vi "Transform.vi"(8 "error in (no error)":errorcluster caption="entrée d'erreur (pas d'erreur)", 9 "y":string[][](array[string]), 10 "X":string[][](array[string]), 11 "KernelCenterer.lvclass":refnum<class "KernelCenterer.lvclass">) -> (0 "error out":errorcluster caption="sortie d'erreur", 2 "Data":T1, 3 "KernelCenterer.lvclass":refnum<class "KernelCenterer.lvclass">)   [LabVIEW 2020, in "KernelCenterer.lvclass"]
doc: "Center kernel matrix.\n\nReturns : \n\n- K_new : numpy array of shape [n_samples1, n_samples2]"
uses:
  KernelCenterer.lvclass
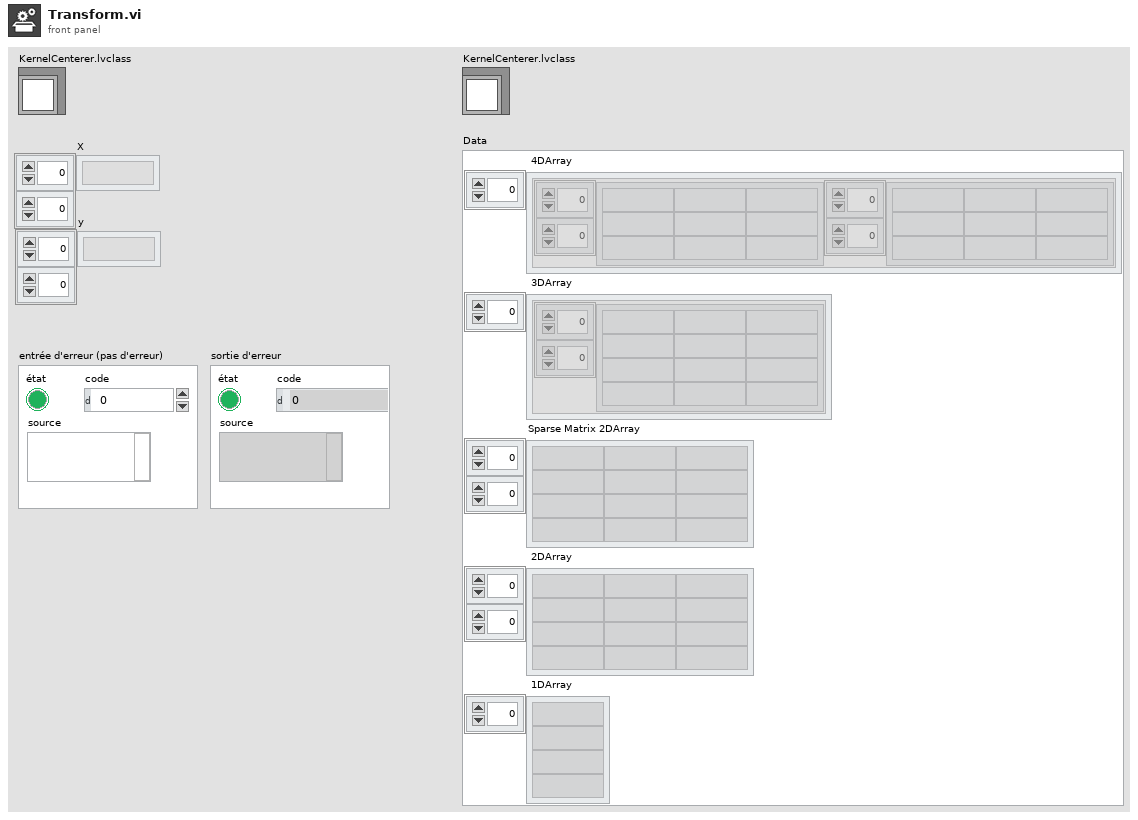
[diagram p1: front panel]
types:
  T1 = cluster{" 4DArray":cluster{"1":string[][], "2":string[][]}[], " 3DArray":cluster{"Tableau":string[][]}[], "Sparse Matrix 2DArray":string[][], " 2DArray":string[][], " 1DArray":string[]}
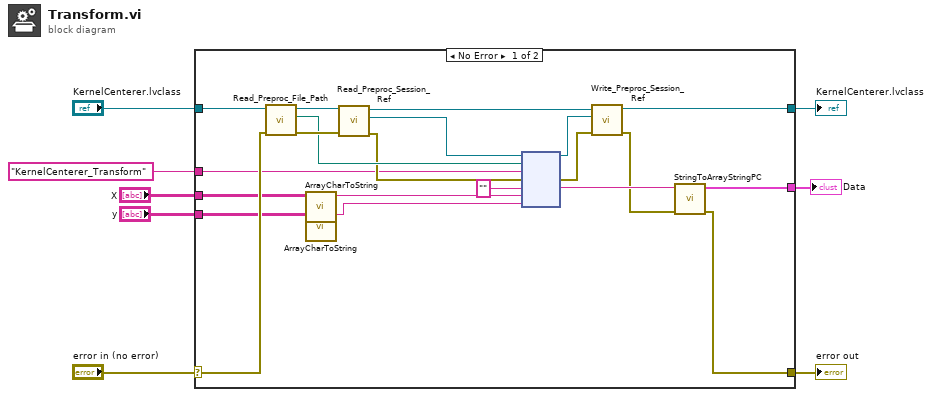
[diagram p0: block diagram]
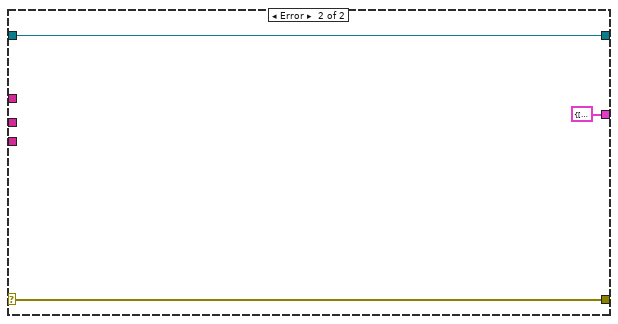
[diagram p2: hidden frame]
diagram:
  n1 = case shown="No Error" "error in (no error)" {
    selector: "error in (no error)" -> [w19 w32]
    tunnel: [w9 w32] -> w7
    tunnel: [w12 w31] -> w5
    tunnel: "KernelCenterer.lvclass" -> [w20 w31]
    tunnel: "KernelCenterer_Transform" ("Fonction") -> [w18 _]
    tunnel: [w10 T1 {" 4DArray"=[], " 3DArray"=[], "Sparse Matrix 2DArray"=[], " 2DArray"=[], " 1DArray"=[]} ("Data")] -> w1
    tunnel: "X" -> [w17 _]
    tunnel: "y" -> [w16 _]
    frame No Error {
      n2 = call-dynamic "Read_Preproc_File_Path.vi"("error in (no error)"=w19, "Python in"=w20) -> ("error out"=w28:errorcluster, "File_Path"=w25:path, "Python out"=w29:refnum<class "KernelCenterer.lvclass">)  [unwired: 7 in]
      n3 = call "ArrayCharToString.vi"("TAB"=w17) -> ("Instruction"=w15:string)  [unwired: 10 in]
      n4 = call "ArrayCharToString.vi"("TAB"=w16) -> ("Instruction"=w14:string)  [unwired: 10 in]
      n5 = call-dynamic "Read_Preproc_Session_Ref.vi"("error in (no error)"=w28, "Python in"=w29) -> ("error out"=w24:errorcluster, "Session_ref"=w26:refnum<k35>, "Python out"=w27:refnum<class "KernelCenterer.lvclass">)  [unwired: 7 in]
      n6 = node(w26, w25, w18, w24, "", w15, w14) -> (w22:refnum<k35>, w23:errorcluster, w13:string)  [unwired: 2 in, 2 out]
      n7 = call-dynamic "Write_Preproc_Session_Ref.vi"("error in (no error)"=w23, "Session_ref"=w22, "Python in"=w27) -> ("error out"=w11:errorcluster, "Python out"=w12:refnum<class "KernelCenterer.lvclass">)  [unwired: 7 in]
      n8 = call "StringToArrayStringPC.vi"("sortie d'erreur"=w11, "Return value"=w13) -> ("sortie d'erreur"=w9:errorcluster, "Data"=w10:T1)  [unwired: 8 in]
    }
    frame Error {
    }
  }
  "error out" <- w7
  "KernelCenterer.lvclass" <- w5
  "Data" <- w1
